vi "appendImage.vi"(8 "error in (no error)":errorcluster, 10 "Image Path":path, 11 "MS-Word in":refnum<class "MS-Word.lvclass">) -> (0 "error out":errorcluster, 3 "MS-Word out":refnum<class "MS-Word.lvclass">)   [LabVIEW 2017, in "LabVIEW NPOI.lvlib" / "MS-Word.lvclass"]
uses:
  MS-Word.lvclass
  MS-Word.lvclass/MS-Word.ctl
  xwpfDocument/xwpfDocument.lvclass
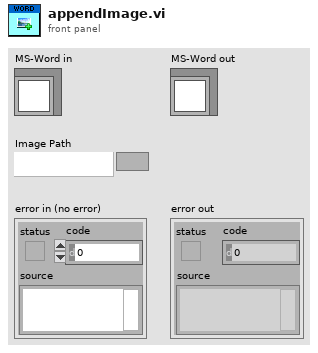
[diagram p1: front panel]
types:
  T1 = enum16{"Title", "Heading 1", "Heading 2", "Heading 3", "Normal", "Figure", "Page Break"}
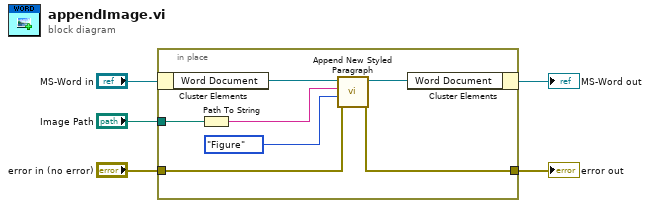
[diagram p0: block diagram]
diagram:
  n1 = in-place {
    in-place-border: "Image Path" -> [w8]
    in-place-border: "error in (no error)" -> [w10]
    in-place-border: [w9] -> w1
    n2 = in-place-cluster #1("MS-Word in") -> ("Word Document"=w12:refnum<class "xwpfDocument.lvclass">)
    n3 = Path To String(path=w8) -> (string=w7:string)
    n4 = call "Append New Styled Paragraph.vi"("error in (no error)"=w10, "Type"=T1."Figure", "Paragraph.Text"=w7, "xwpfDocument in"=w12) -> ("error out"=w9:errorcluster, "xwpfDocument out"=w11:refnum<class "xwpfDocument.lvclass">)  [unwired: 6 in]
    n5 = in-place-cluster #1("Word Document"=w11) -> (→"MS-Word out":refnum<class "MS-Word.lvclass">)
  }
  "error out" <- w1
